vi "EE_Filter_DC_Offset.vi"(4 "Initialiaze?":bool, 7 "Raw Data In":dbl[][](array[numeric])) -> (3 "Filtered Data out":dbl[][](array[numeric]))   [LabVIEW 2016, in "Emotiv Epoc.lvlib"]
uses:
  <vilib>/Analysis/baseanly.llb/Mean (DBL).vi
  Emotiv Epoc.lvlib
  <vilib>/Analysis/NI_AALBase.lvlib
panel:
  # "This VI is a part of BCI Design library, http://www.ru-bci.org \nCopyright © 2020, Sotnikov Peter, All rights reserved. License: GNU GPLv3"
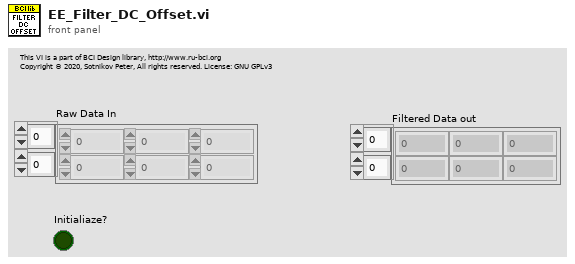
[diagram p1: front panel]
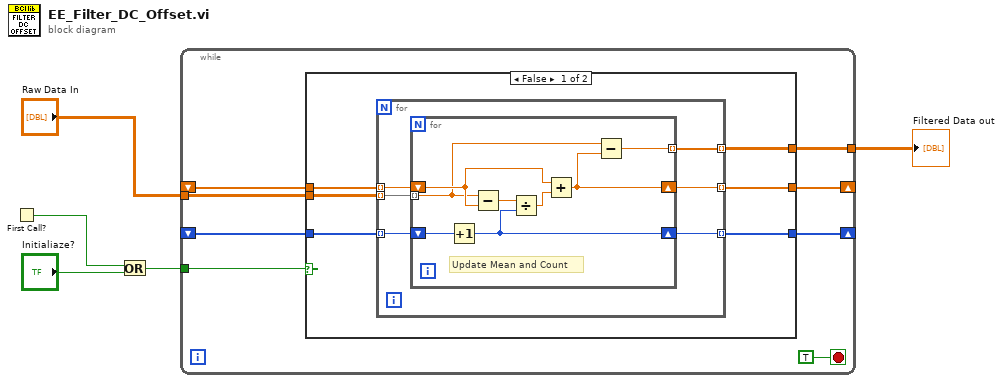
[diagram p0: block diagram]
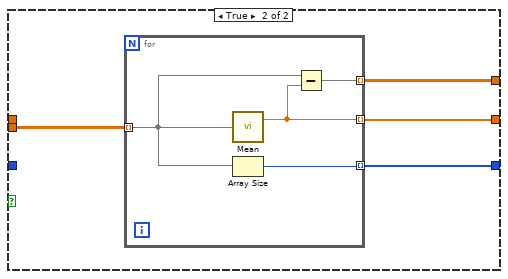
[diagram p2: hidden frame]
diagram:
  n1 = First Call?() -> (First Call?: T/F=w3:bool)
  n2 = Or(x=w3, y="Initialiaze?") -> (x .or. y?=w1:bool)
  n3 = while {
    tunnel: w1 -> [w13]
    tunnel: "Raw Data In" -> [w12]
    shift-right: [w11] -> _
    shift-left: _ -> [w9]
    shift-right: [w10] -> _
    shift-left: _ -> [w8]
    tunnel: [w7] -> w4
    stop <- TRUE stop-if-true
    n4 = case shown="False" w13 {
      tunnel: w12 -> [w18 w37]
      tunnel: [w16 w36] -> w11
      tunnel: [w15 w35] -> w10
      tunnel: w9 -> [w19 _]
      tunnel: w8 -> [w17 _]
      tunnel: [w14 w34] -> w7
      frame False {
        n5 = for {
          tunnel: w19 -> [w23] mode=indexing
          tunnel: w18 -> [w25] mode=indexing
          tunnel: w17 -> [w24] mode=indexing
          tunnel: [w22] -> w16 mode=indexing
          tunnel: [w21] -> w15 mode=indexing
          tunnel: [w20] -> w14 mode=indexing
          n6 = for {
            tunnel: w25 -> [w28] mode=indexing
            shift-right: [w27] -> w22
            shift-left: w23 -> [w30]
            shift-right: [w29] -> w21
            shift-left: w24 -> [w33]
            tunnel: [w26] -> w20 mode=indexing
            # "Update Mean and Count"
            n7 = Increment(x=w33) -> (x+1=w29:i32)
            n8 = Subtract(x=w28, y=w30) -> (x-y=w32:dbl)
            n9 = Divide(x=w32, y=w29) -> (x/y=w31:dbl)
            n10 = Add(x=w30, y=w31) -> (x+y=w27:dbl)
            n11 = Subtract(x=w28, y=w27) -> (x-y=w26:dbl)
          }
        }
      }
      frame True {
        n12 = for {
          tunnel: w37 -> [w40] mode=indexing
          tunnel: [w39] -> w36 mode=indexing
          tunnel: [w41] -> w35 mode=indexing
          tunnel: [w38] -> w34 mode=indexing
          n13 = call-poly <vilib>:"Mean.vi"("X"=w40) -> ("mean"=w39:dbl)  [unwired: 1 out]
          n14 = Array Size(array=w40) -> (size(s)=w41:i32)
          n15 = Subtract(x=w40, y=w39) -> (x-y=w38:dbl[])
        }
      }
    }
  }
  "Filtered Data out" <- w4
